vi "ComicCleaner_SM.vi"() -> ()   [LabVIEW 2023]
uses:
  <vilib>/Utility/config.llb/Write Key (Boolean).vi
  <userlib>/_OpenG.lib/array/array.llb/Remove Duplicates from 1D Array (String)__ogtk.vi
  <userlib>/_OpenG.lib/file/file.llb/Strip Path Extension - String__ogtk.vi
  <userlib>/_OpenG.lib/file/file.llb/Convert File Extension (Path)__ogtk.vi
  <vilib>/Utility/config.llb/NI_LVConfig.lvlib
panel:
  out "Destination":string
  out "Working Folder":path
  in  "Clean":bool
  in  "Clean Filename":bool=TRUE
  out "Crufted Files":string
  out "File List":string
  in  "File Path":path
  out "status":string
  in  "Quit":bool
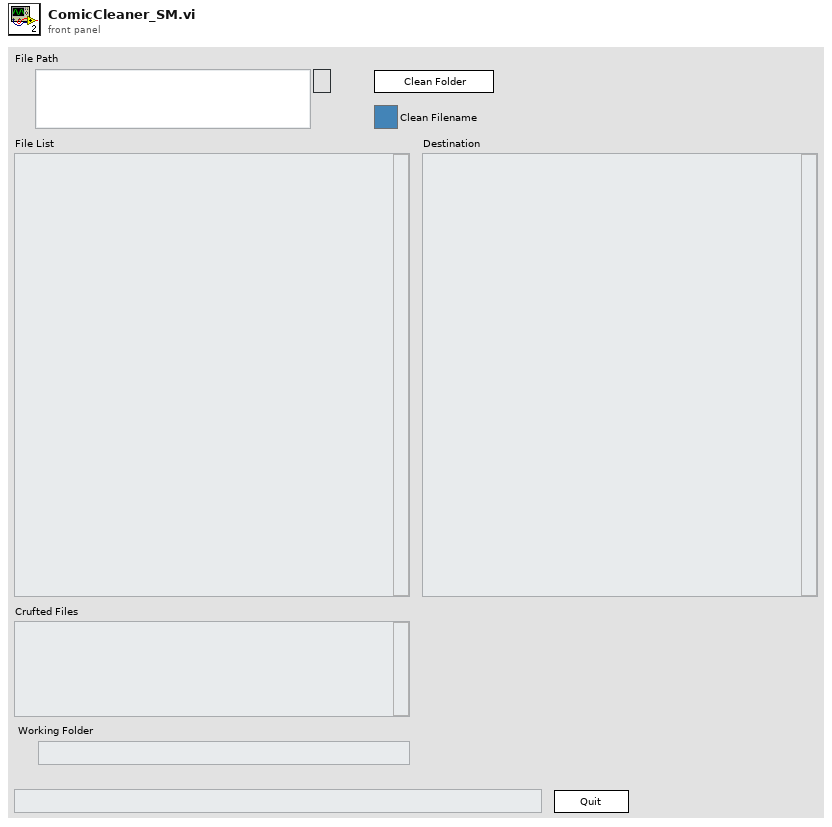
[diagram p1: front panel]
types:
  T1 = enum32{"Invalid", "Standard", "Closed", "Hidden", "Minimized", "Maximized"}
  T2 = enum32{"invalid app kind", "Development System", "Run Time System", "Student Edition", "Embedded LabVIEW", "Evaluation", "Custom"}
  T3 = enum8{"Enabled", "Disabled", "Disabled and Grayed Out"}
  T4 = cluster{"Core":cluster{"Current VI Reference":refnum<vi>, "Close Panel on Exit?":bool}, "Working Folder":path, "Known Tags":set{string}, "ini path":path, "files":path[], "current file index":i32, "deleted filenames":string[], "known found":bool, "abort":bool}
  T5 = cluster{"Current VI Reference":refnum<vi>, "Close Panel on Exit?":bool}
  T6 = typedef "NI_LVConfig.lvlib/Config Data RefNum.ctl" = refnum<k1>
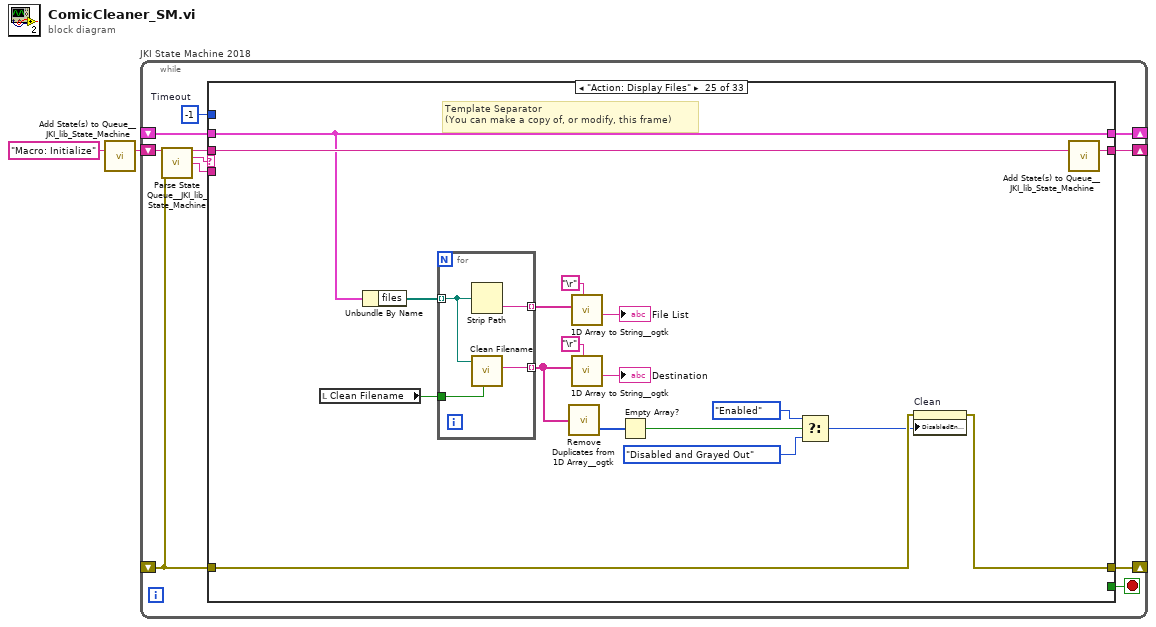
[diagram p0: block diagram]
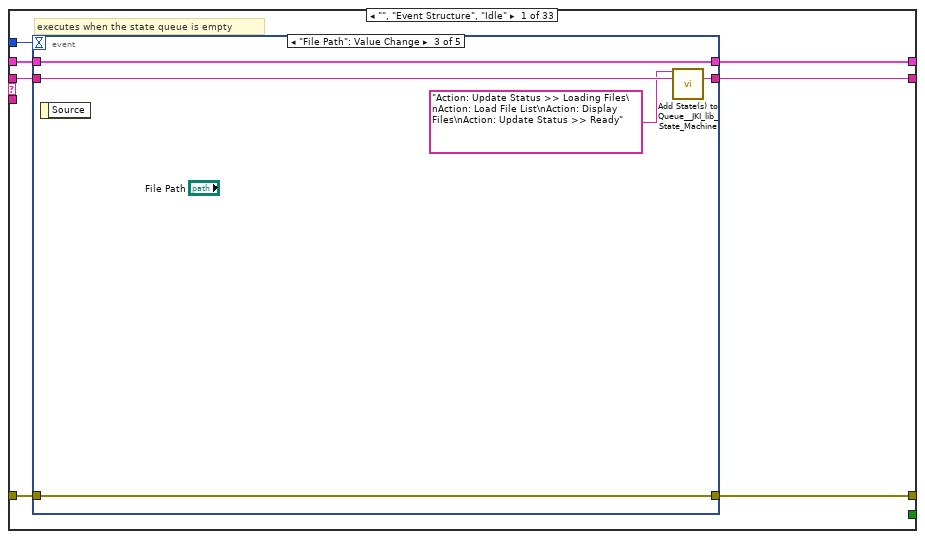
[diagram p2: hidden frame]
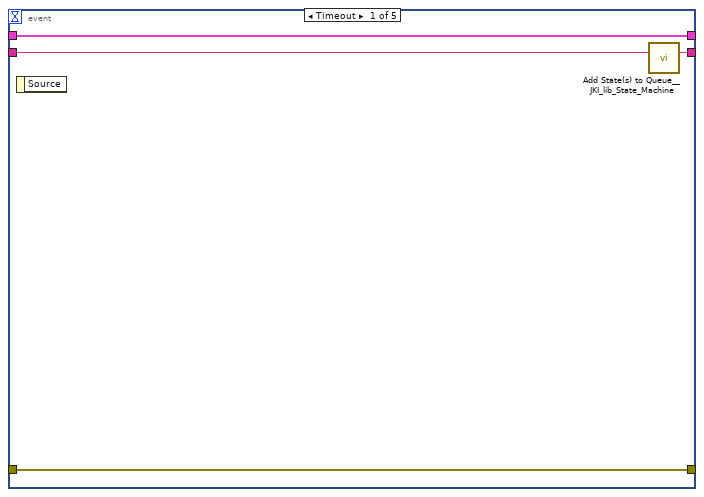
[diagram p3: hidden frame]
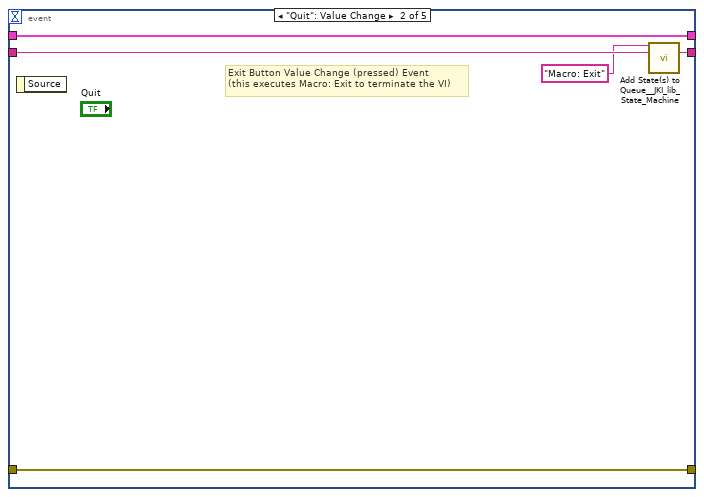
[diagram p4: hidden frame]
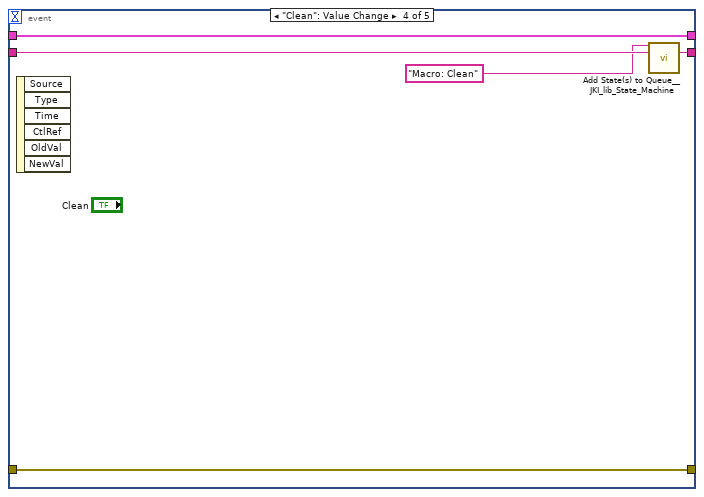
[diagram p5: hidden frame]
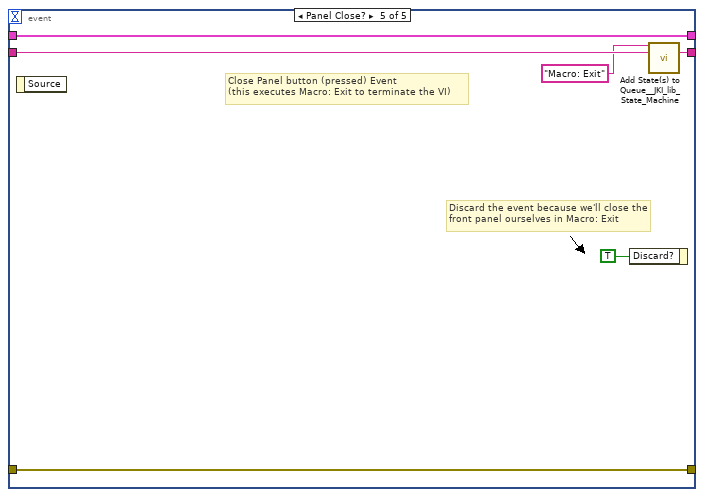
[diagram p6: hidden frame]
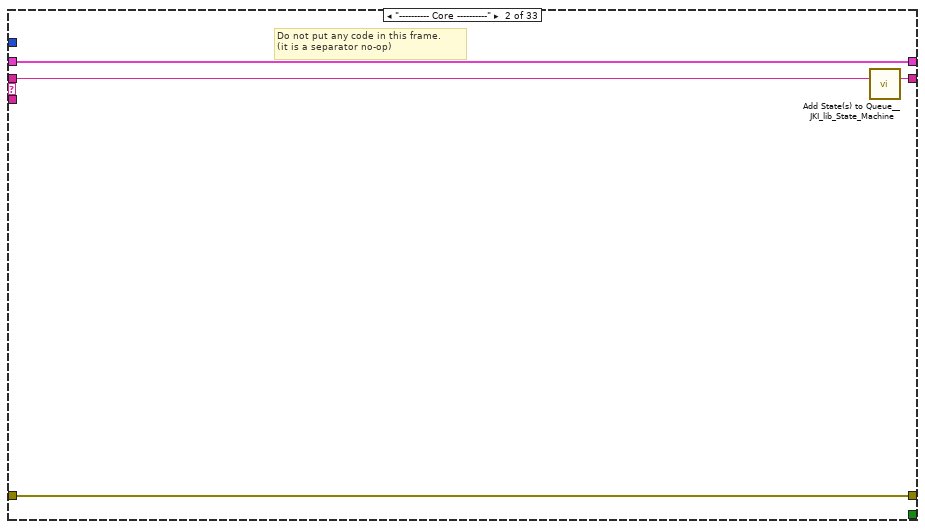
[diagram p7: hidden frame]
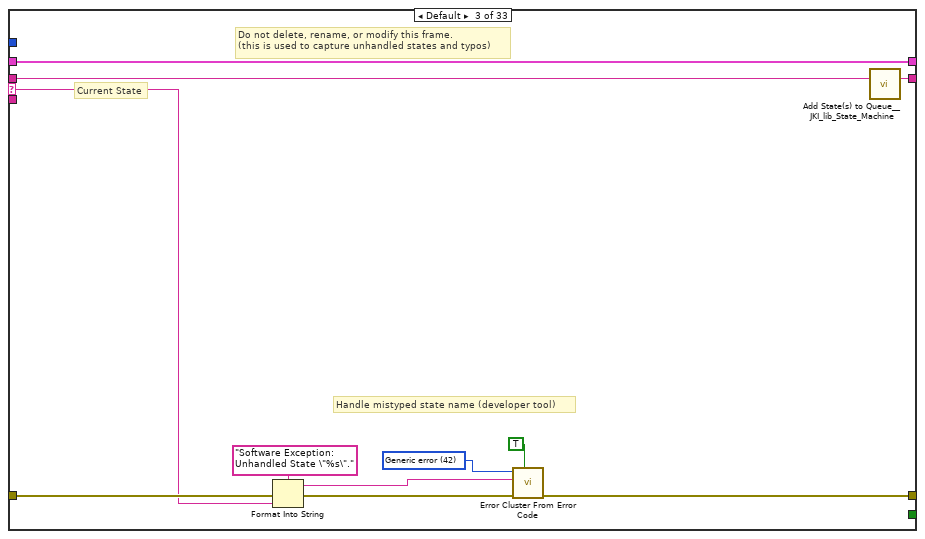
[diagram p8: hidden frame]
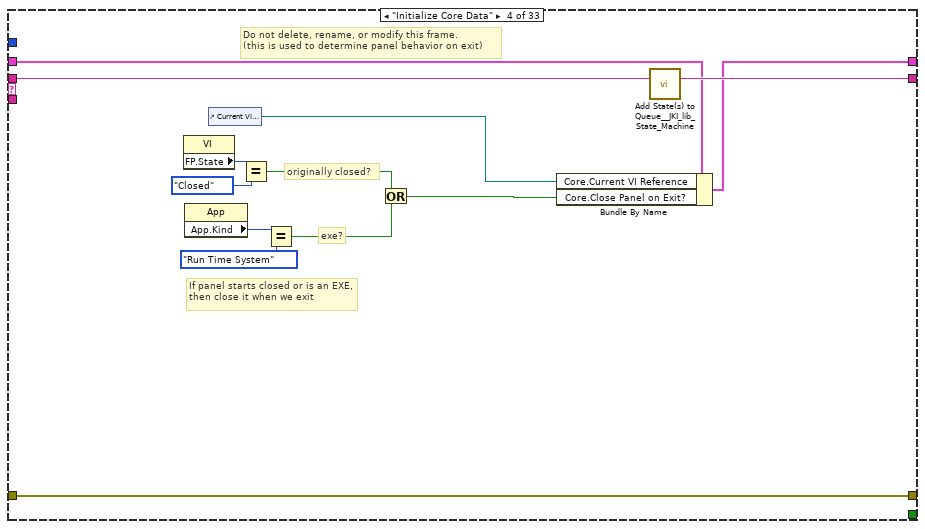
[diagram p9: hidden frame]
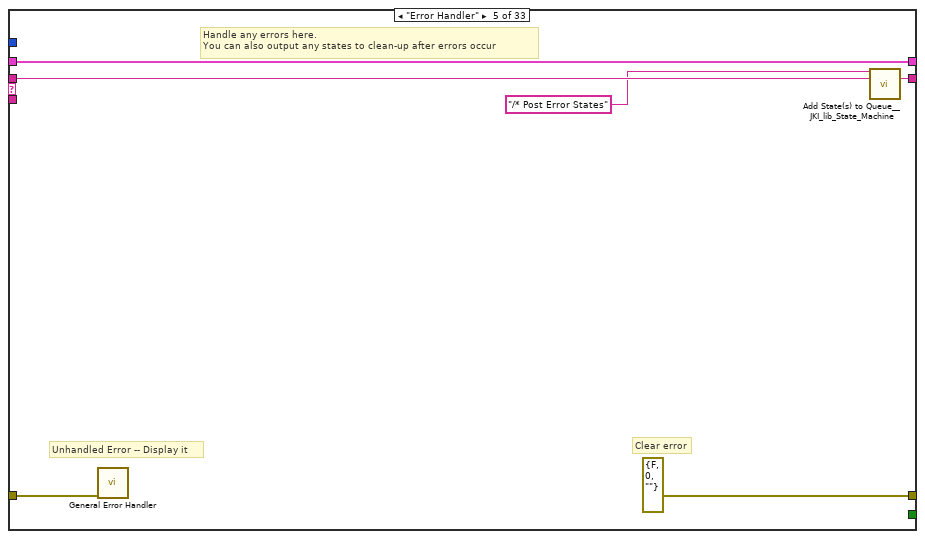
[diagram p10: hidden frame]
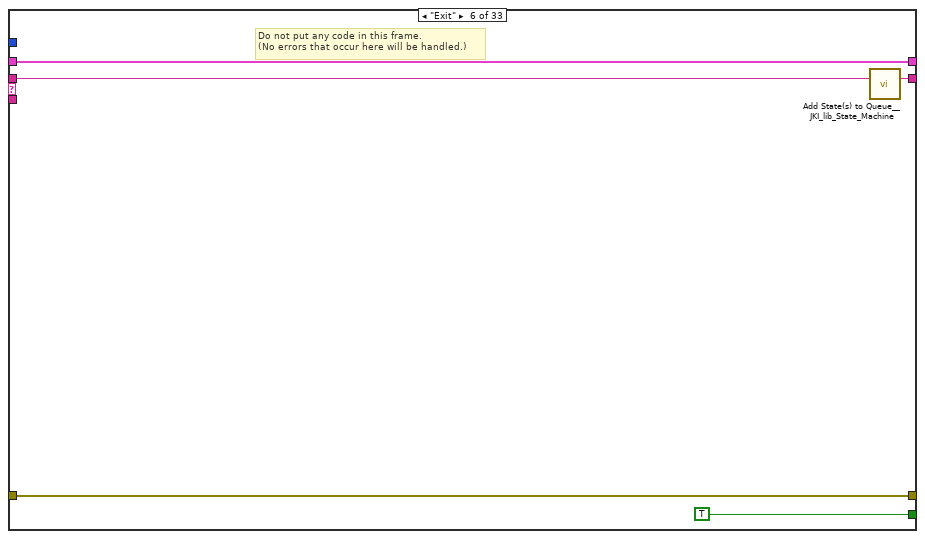
[diagram p11: hidden frame]
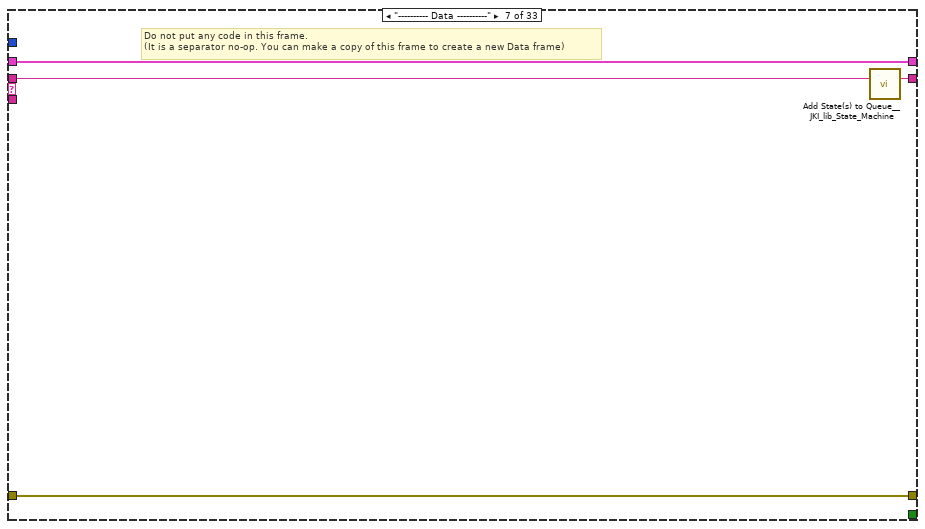
[diagram p12: hidden frame]
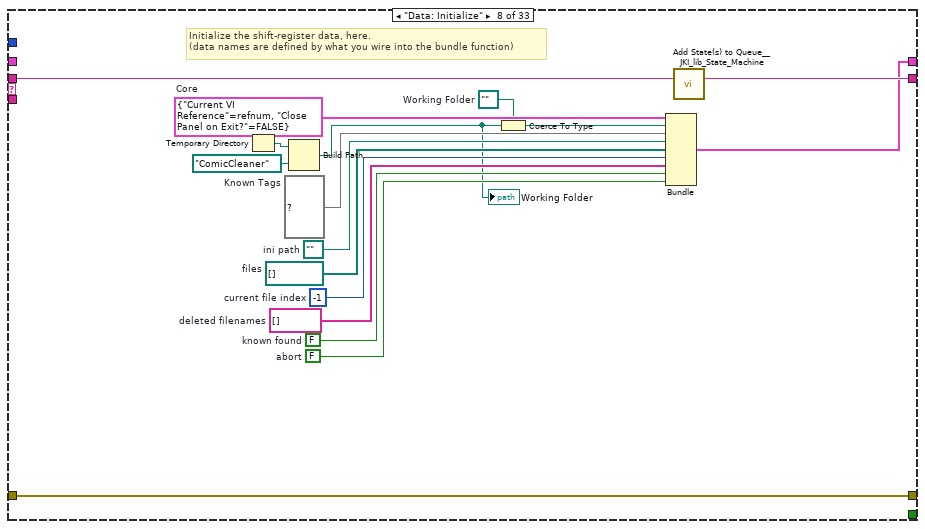
[diagram p13: hidden frame]
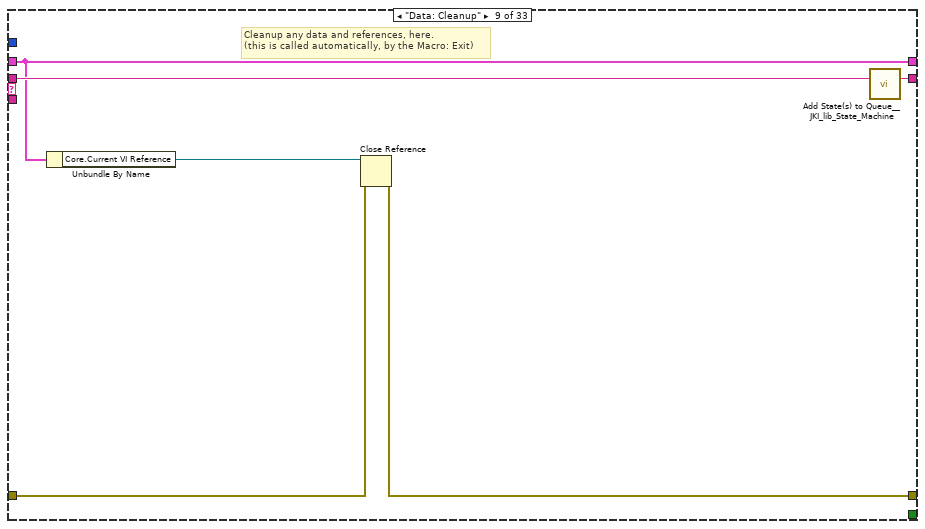
[diagram p14: hidden frame]
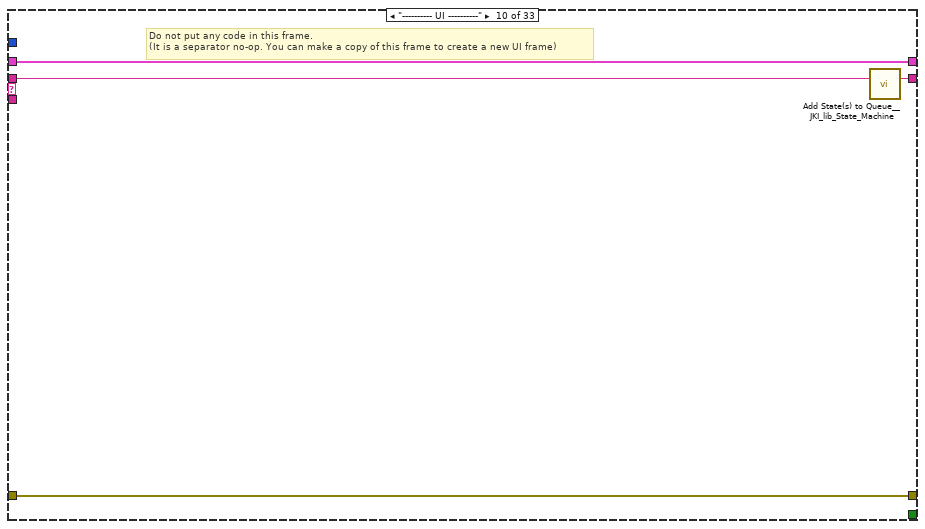
[diagram p15: hidden frame]
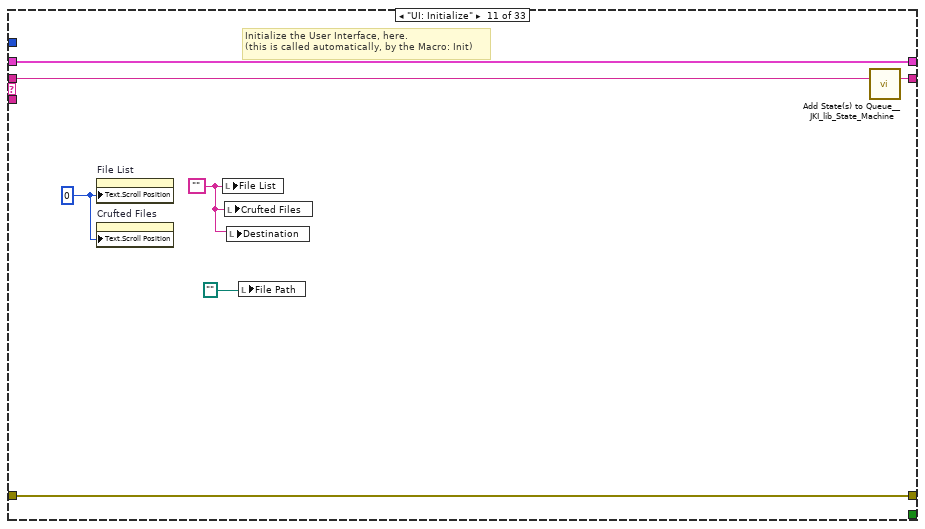
[diagram p16: hidden frame]
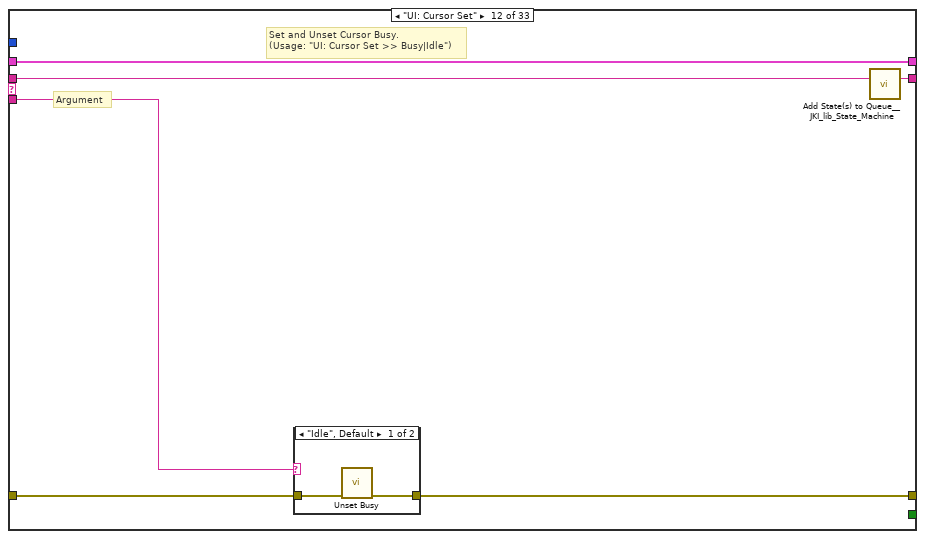
[diagram p17: hidden frame]
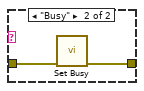
[diagram p18: hidden frame]
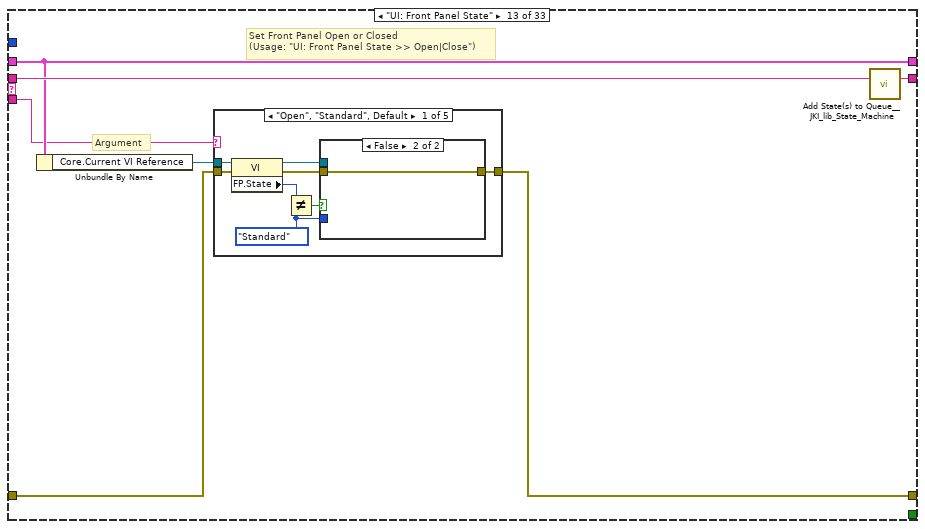
[diagram p19: hidden frame]
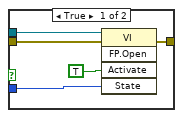
[diagram p20: hidden frame]
diagram:
  n1 = call <vilib>:"Add State(s) to Queue__JKI_lib_State_Machine.vi"("State(s) in (\"\")"="Macro: Initialize") -> ("States Out"=w2:string)  [unwired: 14 in]
  n2 = while "JKI State Machine 2018" {
    shift-right: [w6] -> _
    shift-left: _ -> [w5]
    shift-right: [w9] -> _
    shift-left: _ -> [w3]
    shift-right: [w8] -> _
    shift-left: w2 -> [w10]
    stop <- w7 stop-if-true
    w4 = -1  # Timeout
    n3 = call <vilib>:"Parse State Queue__JKI_lib_State_Machine.vi"("State Queue"=w10, "Error In (no error)"=w3) -> ("Remaining States"=w12:string, "Current State"=w13:string, "Arguments"=w11:string)  [unwired: 11 in]
    n4 = case shown="\"Action: Display Files\"" w13 {
      selector: w13 -> [_ _ w50 _ _ _ _ _ _ _ _ _ _ _ _ _ _ _ _ _ _ _ _ _ _ _ _ _ _ _ _ _ _]
      tunnel: w12 -> [w20 w49 w54 w73 w79 w84 w88 w105 w111 w115 w122 w128 w139 w208 w217 w239 w249 w253 w257 w267 w288 w307 w312 w325 w353 w361 w378 w388 w411 w433 w472 w508 w566]
      tunnel: w11 -> [_ _ _ _ _ _ _ _ _ _ _ w123 w133 _ _ _ _ _ _ _ _ w296 w308 _ _ _ _ _ _ _ _ _ _]
      tunnel: w5 -> [w18 w46 w52 w66 w76 w82 w85 _ w106 w112 w120 w126 w135 w205 w211 w236 w246 w250 w254 w259 w276 w304 w309 w319 w351 w358 w364 w381 w404 w427 w462 w496 w542]
      tunnel: [w17 w47 w56 w70 errorcluster {"status"=FALSE, "code"=0, "source"=""} ("error out") w81 w86 w102 w107 w113 w119 w124 w136 w206 w215 w237 w247 w251 w255 w260 w272 w292 w310 w314 w340 w359 w362 w379 w402 w428 w463 w499 w544] -> w9
      tunnel: w3 -> [w16 w47 w55 w70 w75 w81 w86 w102 w108 w113 w119 w125 w137 w206 w215 w237 w247 w251 w255 w265 w271 w293 w310 w320 w341 w359 w363 w380 w403 w429 w469 w504 w562]
      tunnel: [w19 w48 w53 w72 w78 w83 w87 w104 w110 w114 w121 w127 w138 w207 w216 w238 w248 w252 w256 w266 w287 w306 w311 w324 w352 w360 w377 w387 w410 w432 w471 w507 w565] -> w8
      tunnel: [_ _ _ _ _ TRUE _ _ _ _ _ _ _ _ _ _ _ _ _ _ _ _ _ _ _ _ _ _ _ _ _ _ _] -> w7
      tunnel: [w15 w46 w52 w71 w76 w82 w85 w103 w106 w112 w120 w126 w135 w205 w210 w236 w246 w250 w254 w259 w275 w305 w309 w318 w351 w358 w364 w381 w404 w426 w461 w494 w541] -> w6
      tunnel: w4 -> [w14 _ _ _ _ _ _ _ _ _ _ _ _ _ _ _ _ _ _ _ _ _ _ _ _ _ _ _ _ _ _ _ _]
      frame "", "Event Structure", "Idle" {
        # "executes when the state queue is empty"
        n5 = event shown="[2] \"File Path\": Value Change" {
          selector: _ -> [_ _ _ _ _]
          dyn-events: _ -> [_ _ _ _ _]
          timeout: w14 -> [_ _ _ _ _]
          tunnel: w20 -> [w24 w29 w34 w39 w45]
          tunnel: [w23 w28 w33 w38 w44] -> w19
          tunnel: w18 -> [w21 w26 w31 w36 w42]
          tunnel: [w22 w27 w32 w37 w43] -> w17
          tunnel: w16 -> [w22 w27 w32 w37 w43]
          tunnel: [w21 w26 w31 w36 w42] -> w15
          event Timeout {
            n6 = event-data() -> ()  [unwired: 1 in, 1 out]
            n7 = call <vilib>:"Add State(s) to Queue__JKI_lib_State_Machine.vi"("State(s) in (\"\")"=w24) -> ("States Out"=w23:string)  [unwired: 14 in]
          }
          event "Quit": Value Change {
            # "Exit Button Value Change (pressed) Event\n(this executes Macro: Exit to terminate the VI)"
            n8 = event-data() -> ()  [unwired: 1 in, 1 out]
            n9 = call <vilib>:"Add State(s) to Queue__JKI_lib_State_Machine.vi"("State(s) in Front (\"\")"="Macro: Exit", "State(s) in (\"\")"=w29) -> ("States Out"=w28:string)  [unwired: 13 in]
          }
          event "File Path": Value Change {
            n10 = event-data() -> ()  [unwired: 1 in, 1 out]
            n11 = call <vilib>:"Add State(s) to Queue__JKI_lib_State_Machine.vi"("State(s) in Front (\"\")"="Action: Update Status >> Loading Files\nAction: Load File List\nAction: Display Files\nAction: Update Status >> Ready", "State(s) in (\"\")"=w34) -> ("States Out"=w33:string)  [unwired: 13 in]
          }
          event "Clean": Value Change {
            n12 = event-data() -> ()  [unwired: 1 in, 6 out]
            n13 = call <vilib>:"Add State(s) to Queue__JKI_lib_State_Machine.vi"("State(s) in Front (\"\")"="Macro: Clean", "State(s) in (\"\")"=w39) -> ("States Out"=w38:string)  [unwired: 13 in]
          }
          event Panel Close? {
            # "Discard the event because we'll close the front panel ourselves in Macro: Exit"
            # "Close Panel button (pressed) Event\n(this executes Macro: Exit to terminate the VI)"
            n14 = event-data() -> ()  [unwired: 1 in, 1 out]
            n15 = event-data("Discard?"=TRUE) -> ()  [unwired: 1 in, 1 out]
            n16 = call <vilib>:"Add State(s) to Queue__JKI_lib_State_Machine.vi"("State(s) in Front (\"\")"="Macro: Exit", "State(s) in (\"\")"=w45) -> ("States Out"=w44:string)  [unwired: 13 in]
          }
        }
      }
      frame "---------- Core ----------" {
        # "Do not put any code in this frame.\n(it is a separator no-op)"
        n17 = call <vilib>:"Add State(s) to Queue__JKI_lib_State_Machine.vi"("State(s) in (\"\")"=w49) -> ("States Out"=w48:string)  [unwired: 14 in]
      }
      frame Default {
        w59 = 42 items=["No error", "Argument error", "Memory is full", "Out of zone", "End of file", "File already open", "Generic file I/O error", "File not found", "File permission error", "Disk is full", "Duplicate path", "Too many files open", "System feature not enabled", "Resource file not found", "Cannot add resource", "Resource not found", "Image not found", "Image memory error", "Pen does not exist", "Config type invalid", "Config token not found", "Config parse error", "Config memory error", "Bad external code format", "Bad external code offset", "External code not present", "Null window", "Destroy window error", "Null menu", "Print aborted", "Bad print record", "Print driver error", "Windows error during printing", "Memory error during printing", "Print dialog error", "Generic print error", "Invalid device refnum", "Device not found", "Device parameter error", "Device unit error", "Cannot open device", "Device call aborted", "Generic error", "Cancelled by user", "Object ID too low", "Object ID too high", "Object not in heap", "Unknown heap", "Unknown object (invalid DefProc)", "Unknown object (DefProc not in table)", "Message out of range", "Invalid (null) method", "Unknown message", "Manager call not supported", "Bad address", "Network operation in progress", "Network operation timed out", "Connection is busy", "Network attribute not supported", "Network error", "Address in use", "System out of memory", "Connection aborted", "Connection refused", "Not connected", "Already connected", "Connection closed", "Initialization error (interapplication manager)", "Bad occurrence", "Wait on unbound occurrence handler", "Occurrence queue overflow", "Datalog type conflict", "Unused", "Unrecognized type (interapplication manager)", "Memory corrupt", "Failed to make temporary DLL", "Old CIN version", "Drag socket not found", "Failed to load drop-object", "Failed to register OLE object", "Failed to release OLE object", "Format specifier type mismatch", "Unknown format specifier", "Too few format specifiers", "Too many format specifiers", "Scan failed", "Newer CIN version", "Error converting to variant", "Runtime menu error", "Password tampered", "Variant attribute not found", "Incompatible variant data type", "Event data is not available", "Event Store is not present", "Occurrence is not found", "Event Queue is not created", "Event info is not available", "Refnum passed is NULL", "Error retrieving Class GUID", "Error retrieving CoClass GUID", "Error retrieving TypeLib GUID.", "Bad built application magic bytes.", "Specific driver is different from the specific driver associated with the Logical Name.", "There is no session opened to the class driver.", "Max Error", "MAX - Error with config objects", "MAX - Error loading configuration", "MAX - Group not supported"]
        # "Current State"
        # "Do not delete, rename, or modify this frame.\n(this is used to capture unhandled states and typos)"
        # "Handle mistyped state name (developer tool)"
        n18 = Format Into String(format string="Software Exception: Unhandled State \"%s\"." ("message"), error in=w55, w50) -> (resulting string=w58:string, error out=w57:errorcluster)  [unwired: 1 in]
        n19 = call <vilib>:"Error Cluster From Error Code.vi"("show call chain? (False)"=TRUE, "error in (no error)"=w57, "error message (\"\")"=w58, "error code (0)"=w59) -> ("error out"=w56:errorcluster)  [unwired: 5 in]
        n20 = call <vilib>:"Add State(s) to Queue__JKI_lib_State_Machine.vi"("State(s) in (\"\")"=w54) -> ("States Out"=w53:string)  [unwired: 14 in]
      }
      frame "Initialize Core Data" {
        # "Do not delete, rename, or modify this frame.\n(this is used to determine panel behavior on exit)"
        # "originally closed?"
        # "exe?"
        # "If panel starts closed or is an EXE, then close it when we exit"
        n21 = property class="VI"() -> ("FP.State"=w63:T1)  [unwired: 2 in, 2 out]
        n22 = property class="App"() -> ("App.Kind"=w69:T2)  [unwired: 2 in, 2 out]
        n23 = control-ref of="Current VI Reference"() -> (w64:refnum<vi>)
        n24 = Equal?(x=w63, y=T1."Closed" ("Front Panel Window:State")) -> (x = y?=w61:bool)
        n25 = Equal?(x=w69, y=T2."Run Time System" ("Application:Kind")) -> (x = y?=w67:bool)
        n26 = Or(x=w61, y=w67) -> (x .or. y?=w65:bool)
        n27 = Bundle By Name(cluster=w66, "Core.Current VI Reference"=w64, "Core.Close Panel on Exit?"=w65) -> (w71:T4)
        n28 = call <vilib>:"Add State(s) to Queue__JKI_lib_State_Machine.vi"("State(s) in (\"\")"=w73) -> ("States Out"=w72:string)  [unwired: 14 in]
      }
      frame "Error Handler" {
        # "Unhandled Error -- Display it"
        # "Handle any errors here.\nYou can also output any states to clean-up after errors occur"
        # "Clear error"
        n29 = call <vilib>:"General Error Handler.vi"("error in (no error)"=w75) -> ()  [unwired: 10 in, 5 out]
        n30 = call <vilib>:"Add State(s) to Queue__JKI_lib_State_Machine.vi"("State(s) in Front (\"\")"="/* Post Error States", "State(s) in (\"\")"=w79) -> ("States Out"=w78:string)  [unwired: 13 in]
      }
      frame "Exit" {
        # "Do not put any code in this frame.\n(No errors that occur here will be handled.)"
        n31 = call <vilib>:"Add State(s) to Queue__JKI_lib_State_Machine.vi"("State(s) in (\"\")"=w84) -> ("States Out"=w83:string)  [unwired: 14 in]
      }
      frame "---------- Data ----------" {
        # "Do not put any code in this frame.\n(It is a separator no-op. You can make a copy of this frame to create a new Data frame)"
        n32 = call <vilib>:"Add State(s) to Queue__JKI_lib_State_Machine.vi"("State(s) in (\"\")"=w88) -> ("States Out"=w87:string)  [unwired: 14 in]
      }
      frame "Data: Initialize" {
        w90 = FALSE  # abort
        w91 = FALSE  # known found
        w92 = string[] []  # deleted filenames
        w93 = -1  # current file index
        w98 = path[] []  # files
        w99 = path ""  # ini path
        w100 = set{string} {}  # Known Tags
        w94 = path ""  # Working Folder
        w101 = T5 {"Current VI Reference"=refnum, "Close Panel on Exit?"=FALSE}  # Core
        # "Initialize the shift-register data, here.\n(data names are defined by what you wire into the bundle function)"
        n33 = Temporary Directory() -> (w97:path)
        n34 = Build Path(base path=w97, name or relative path=path "ComicCleaner") -> (appended path=w89:path)
        "Working Folder" <- w89
        n35 = Coerce To Type(0:w89, 1:w94) -> (2:w95:path)
        n36 = Bundle("Core"=w101, "Working Folder"=w95, "Known Tags"=w100, "ini path"=w99, "files"=w98, "current file index"=w93, "deleted filenames"=w92, "known found"=w91, "abort"=w90) -> (w103:T4)  [unwired: 1 in]
        n37 = call <vilib>:"Add State(s) to Queue__JKI_lib_State_Machine.vi"("State(s) in (\"\")"=w105) -> ("States Out"=w104:string)  [unwired: 14 in]
      }
      frame "Data: Cleanup" {
        # "Cleanup any data and references, here.\n(this is called automatically, by the Macro: Exit)"
        n38 = Unbundle By Name(w106) -> ("Core.Current VI Reference"=w109:refnum<vi>)
        n39 = Close Reference(reference=w109, error in (no error)=w108) -> (error out=w107:errorcluster)
        n40 = call <vilib>:"Add State(s) to Queue__JKI_lib_State_Machine.vi"("State(s) in (\"\")"=w111) -> ("States Out"=w110:string)  [unwired: 14 in]
      }
      frame "---------- UI ----------" {
        # "Do not put any code in this frame.\n(It is a separator no-op. You can make a copy of this frame to create a new UI frame)"
        n41 = call <vilib>:"Add State(s) to Queue__JKI_lib_State_Machine.vi"("State(s) in (\"\")"=w115) -> ("States Out"=w114:string)  [unwired: 14 in]
      }
      frame "UI: Initialize" {
        w118 = u32 0 ("Text.Scroll Position")
        w116 = ""
        # "Initialize the User Interface, here.\n(this is called automatically, by the Macro: Init)"
        n42 = property on="File List" class="Str"("Text.Scroll Position"=w118) -> ()  [unwired: 2 in, 2 out]
        n43 = property on="Crufted Files" class="Str"("Text.Scroll Position"=w118) -> ()  [unwired: 2 in, 2 out]
        n44 = local write "File List"(w116) -> ()
        n45 = local write "Crufted Files"(w116) -> ()
        n46 = local write "Destination"(w116) -> ()
        n47 = local write "File Path"(path "") -> ()
        n48 = call <vilib>:"Add State(s) to Queue__JKI_lib_State_Machine.vi"("State(s) in (\"\")"=w122) -> ("States Out"=w121:string)  [unwired: 14 in]
      }
      frame "UI: Cursor Set" {
        # "Argument"
        # "Set and Unset Cursor Busy.\n(Usage: \"UI: Cursor Set >> Busy|Idle\")"
        n49 = case shown="\"Idle\", Default" w123 {
          tunnel: w125 -> [w130 w132]
          tunnel: [w129 w131] -> w124
          frame "Idle", Default {
            n50 = call <vilib>:"Unset Busy.vi"("error in (no error)"=w130) -> ("error out"=w129:errorcluster)  [unwired: 10 in]
          }
          frame "Busy" {
            n51 = call <vilib>:"Set Busy.vi"("error in (no error)"=w132) -> ("error out"=w131:errorcluster)  [unwired: 9 in, 1 out]
          }
        }
        n52 = call <vilib>:"Add State(s) to Queue__JKI_lib_State_Machine.vi"("State(s) in (\"\")"=w128) -> ("States Out"=w127:string)  [unwired: 14 in]
      }
      frame "UI: Front Panel State" {
        # "Argument"
        # "Set Front Panel Open or Closed\n(Usage: \"UI: Front Panel State >> Open|Close\")"
        n53 = Unbundle By Name(w135) -> ("Core.Current VI Reference"=w134:refnum<vi>)
        n54 = case shown="\"Open\", \"Standard\", Default" w133 {
          tunnel: w137 -> [w145 w160 w171 w184 w197]
          tunnel: [w147 w161 w173 w186 w199] -> w136
          tunnel: w134 -> [w146 w158 w172 w185 w198]
          frame "Open", "Standard", Default {
            w140 = T1."Standard" ("State")
            n55 = property class="VI"(reference=w146, error in=w145) -> (reference out=w143:refnum<vi>, error out=w144:errorcluster, "FP.State"=w142:T1)
            n56 = Not Equal?(x=w142, y=w140) -> (x != y?=w141:bool)
            n57 = case shown="False" w141 {
              tunnel: [w151 w153] -> w147
              tunnel: w144 -> [w150 w153]
              tunnel: w143 -> [w149 _]
              tunnel: w140 -> [w148 _]
              frame True {
                n58 = invoke class="VI" method="FP.Open"(reference=w149, error in=w150, "Activate"=TRUE, "State"=w148) -> (error out=w151:errorcluster)  [unwired: 1 in, 4 out]
              }
              frame False {
              }
            }
          }
          frame "Close", "Closed" {
            n59 = property class="VI"(reference=w158, error in=w160) -> (reference out=w157:refnum<vi>, error out=w159:errorcluster, "FP.State"=w155:T1)
            n60 = Not Equal?(x=w155, y=T1."Closed" ("Front Panel Window:State")) -> (x != y?=w154:bool)
            n61 = case shown="True" w154 {
              tunnel: [w162 w165] -> w161
              tunnel: w159 -> [w162 w164]
              tunnel: w157 -> [_ w163]
              frame False {
              }
              frame True {
                n62 = invoke class="VI" method="FP.Close"(reference=w163, error in=w164) -> (error out=w165:errorcluster)  [unwired: 1 in, 2 out]
              }
            }
          }
          frame "Hidden", "Hide" {
            w166 = T1."Hidden" ("State")
            n63 = property class="VI"(reference=w172, error in=w171) -> (reference out=w169:refnum<vi>, error out=w170:errorcluster, "FP.State"=w168:T1)
            n64 = Not Equal?(x=w168, y=w166) -> (x != y?=w167:bool)
            n65 = case shown="True" w167 {
              tunnel: [w177 w178] -> w173
              tunnel: w170 -> [w176 w178]
              tunnel: w169 -> [w175 _]
              tunnel: w166 -> [w174 _]
              frame True {
                n66 = invoke class="VI" method="FP.Open"(reference=w175, error in=w176, "State"=w174) -> (error out=w177:errorcluster)  [unwired: 2 in, 4 out]
              }
              frame False {
              }
            }
          }
          frame "Minimize", "Minimized" {
            w179 = T1."Minimized" ("State")
            n67 = property class="VI"(reference=w185, error in=w184) -> (reference out=w182:refnum<vi>, error out=w183:errorcluster, "FP.State"=w181:T1)
            n68 = Not Equal?(x=w181, y=w179) -> (x != y?=w180:bool)
            n69 = case shown="True" w180 {
              tunnel: [w190 w191] -> w186
              tunnel: w183 -> [w189 w191]
              tunnel: w182 -> [w188 _]
              tunnel: w179 -> [w187 _]
              frame True {
                n70 = invoke class="VI" method="FP.Open"(reference=w188, error in=w189, "State"=w187) -> (error out=w190:errorcluster)  [unwired: 2 in, 4 out]
              }
              frame False {
              }
            }
          }
          frame "Maximize", "Maximized" {
            w192 = T1."Maximized" ("State")
            n71 = property class="VI"(reference=w198, error in=w197) -> (reference out=w195:refnum<vi>, error out=w196:errorcluster, "FP.State"=w194:T1)
            n72 = Not Equal?(x=w194, y=w192) -> (x != y?=w193:bool)
            n73 = case shown="True" w193 {
              tunnel: [w203 w204] -> w199
              tunnel: w196 -> [w202 w204]
              tunnel: w195 -> [w201 _]
              tunnel: w192 -> [w200 _]
              frame True {
                n74 = invoke class="VI" method="FP.Open"(reference=w201, error in=w202, "State"=w200) -> (error out=w203:errorcluster)  [unwired: 2 in, 4 out]
              }
              frame False {
              }
            }
          }
        }
        n75 = call <vilib>:"Add State(s) to Queue__JKI_lib_State_Machine.vi"("State(s) in (\"\")"=w139) -> ("States Out"=w138:string)  [unwired: 14 in]
      }
      frame "---------- Macro ----------" {
        # "Do not put any code in this frame.\n(It is a separator no-op. You can make a copy of this frame to create a new Macro frame)"
        n76 = call <vilib>:"Add State(s) to Queue__JKI_lib_State_Machine.vi"("State(s) in (\"\")"=w208) -> ("States Out"=w207:string)  [unwired: 14 in]
      }
      frame "Macro: Clean" {
        n77 = Unbundle By Name(w211) -> ("files"=w213:path[], "current file index"=w212:i32, "abort"=w214:bool)
        n78 = case shown="False" w214 {
          tunnel: w213 -> [w225 _]
          tunnel: w212 -> [w224 _]
          tunnel: w211 -> [w221 w234]
          tunnel: [w219 w234] -> w210
          tunnel: [w218 _] -> w209
          frame False {
            n79 = Array Size(array=w225) -> (size(s)=w223:i32)
            n80 = Increment(x=w224) -> (x+1=w220:i32)
            n81 = Equal?(x=w223, y=w220) -> (x = y?=w222:bool)
            n82 = case shown="False" w222 {
              tunnel: w221 -> [w229 w232]
              tunnel: w220 -> [w228 _]
              tunnel: [w227 w230] -> w219
              tunnel: ["Action: Clean Working Folder\nAction: Update Status >> Expanding Comic\nClean: Expand Comic\nAction: Update Status >> Removing Empty Folders\nClean: Remove Empty Folders\nAction: Update Status >> Resetting Permissions\nClean: Reset Permissions\nAction: Update Status >> Removing Cruft\nClean: Remove Cruft\nAction: Update Status >> Removing Known\nClean: Remove Known\nAction: Update Status >> Removing Unknown\nClean: Clean Unknown\nAction: Update Status >> Compressing Comic\nClean: Compress Comic\nAction: Display Files\nMacro: Clean" "Action: Update Status >> Clean operation complete. Ready"] -> w218
              frame False {
                n83 = Bundle By Name(cluster=w229, "current file index"=w228) -> (w227:T4)
              }
              frame True {
                n84 = Bundle By Name(cluster=w232, "current file index"=-1) -> (w230:T4)
              }
            }
          }
          frame True {
          }
        }
        n85 = call <vilib>:"Add State(s) to Queue__JKI_lib_State_Machine.vi"("State(s) in Front (\"\")"=w209, "State(s) in (\"\")"=w217) -> ("States Out"=w216:string)  [unwired: 13 in]
      }
      frame "Macro: Initialize" {
        # "Initialization Macro\n(This is called once, when the VI starts)"
        n86 = call <vilib>:"Add State(s) to Queue__JKI_lib_State_Machine.vi"("State(s) in Front (\"\")"="Data: Initialize\nInitialize Core Data\nUI: Initialize\nUI: Front Panel State >> Open\nAction: Update Status >> Reading Known Tags\nAction: Read Known Tags\nAction: Update Status >> Cleaning Working Directory\nAction: Clean Working Folder\nAction: Update Status >> Ready", "State(s) in (\"\")"=w239) -> ("States Out"=w238:string)  [unwired: 13 in]
      }
      frame "Macro: Exit" {
        # "Exit Macro\n(This is called once, when the VI exits)"
        n87 = Unbundle By Name(w246) -> ("Core.Close Panel on Exit?"=w245:bool)
        n88 = Select(t="UI: Front Panel State >> Close", s=w245, f="") -> (s? t:f=w242:string)
        n89 = call <vilib>:"Add State(s) to Queue__JKI_lib_State_Machine.vi"("State(s) in (\"\")"=w242, "State(s) at Back (\"\")"="Data: Cleanup\nExit") -> ("States Out"=w240:string)  [unwired: 13 in]
        n90 = call <vilib>:"Add State(s) to Queue__JKI_lib_State_Machine.vi"("State(s) in Front (\"\")"=w240, "State(s) in (\"\")"=w249) -> ("States Out"=w248:string)  [unwired: 13 in]
      }
      frame "Macro: Abort" {
        n91 = call <vilib>:"Add State(s) to Queue__JKI_lib_State_Machine.vi"("State(s) in (\"\")"=w253) -> ("States Out"=w252:string)  [unwired: 14 in]
      }
      frame "---------- Action ----------" {
        # "Template Separator\n(You can make a copy of, or modify, this frame)"
        n92 = call <vilib>:"Add State(s) to Queue__JKI_lib_State_Machine.vi"("State(s) in (\"\")"=w257) -> ("States Out"=w256:string)  [unwired: 14 in]
      }
      frame "Action: Clean Working Folder" {
        n93 = Unbundle By Name(w259) -> ("Working Folder"=w258:path)
        n94 = call <userlib>:"Create Dir if Non-Existant__ogtk.vi"("error in (no error)"=w265, "Directory Path"=w258) -> ("error out"=w261:errorcluster, "dup Directory Path"=w262:path)  [unwired: 7 in, 1 out]
        n95 = call <vilib>:"Recursive File List.vi"("error in (no error)"=w261, "Folder Path"=w262) -> ("error out"=w264:errorcluster, "All Files in Dir"=w263:path[])  [unwired: 5 in, 3 out]
        n96 = for {
          tunnel: w263 -> [w270] mode=indexing
          shift-right: [w268] -> w260
          shift-left: w264 -> [w269]
          n97 = Delete(path (use dialog)=w270, error in=w269) -> (error out=w268:errorcluster)  [unwired: 3 in, 2 out]
        }
        n98 = call <vilib>:"Add State(s) to Queue__JKI_lib_State_Machine.vi"("State(s) in (\"\")"=w267) -> ("States Out"=w266:string)  [unwired: 14 in]
      }
      frame "Action: Read Known Tags" {
        w285 = set{string} {}  # Size: 0
        n99 = Current VI's Path() -> (path=w278:path)
        n100 = Build Path(base path=w278, name or relative path=path "../Comic Cleaner.ini") -> (appended path=w273:path)
        n101 = call <vilib>:"Open Config Data.vi"("error in (no error)"=w271, "configuration file path"=w273) -> ("error out"=w279:errorcluster, "refnum"=w280:T6)  [unwired: 7 in, 1 out]
        n102 = call <vilib>:"Get Key Names.vi"("section"="KnownTags", "error in (no error)"=w279, "refnum"=w280) -> ("error out"=w282:errorcluster, "key names"=w284:string[], "refnum out"=w281:T6)  [unwired: 5 in, 1 out]
        n103 = To Lower Case(string=w284) -> (all lower case string=w286:string[])
        n104 = call <vilib>:"Close Config Data.vi"("error in (no error)"=w282, "refnum"=w281) -> ("error out"=w272:errorcluster)  [unwired: 8 in, 1 out]
        n105 = for {
          shift-right: [w291] -> w274
          shift-left: w285 -> [w290]
          tunnel: w286 -> [w289] mode=indexing
          n106 = Insert Into Set(10:w289, 11:w290) -> (3:w291:set{string})  [unwired: 1 out]
        }
        n107 = Bundle By Name(cluster=w276, "Known Tags"=w274, "ini path"=w273) -> (w275:T4)
        n108 = call <vilib>:"Add State(s) to Queue__JKI_lib_State_Machine.vi"("State(s) in (\"\")"=w288) -> ("States Out"=w287:string)  [unwired: 14 in]
      }
      frame "Action: Add Known Tag" {
        n109 = Unbundle By Name(w304) -> ("Known Tags"=w298:set{string}, "ini path"=w294:path)
        n110 = call <vilib>:"Open Config Data.vi"("error in (no error)"=w293, "configuration file path"=w294) -> ("error out"=w299:errorcluster, "refnum"=w300:T6)  [unwired: 7 in, 1 out]
        n111 = call-poly <vilib>:"Write Key.vi"("section"="KnownTags", "error in (no error)"=w299, "value"=TRUE, "key"=w296, "refnum"=w300) -> ("error out"=w302:errorcluster, "refnum out"=w303:T6)  [unwired: 4 in, 1 out]
        n112 = Insert Into Set(10:w296, 11:w298) -> (3:w297:set{string})  [unwired: 1 out]
        n113 = Bundle By Name(cluster=w304, "Known Tags"=w297) -> (w305:T4)
        n114 = call <vilib>:"Close Config Data.vi"("error in (no error)"=w302, "refnum"=w303) -> ("error out"=w292:errorcluster)  [unwired: 8 in, 1 out]
        n115 = call <vilib>:"Add State(s) to Queue__JKI_lib_State_Machine.vi"("State(s) in (\"\")"=w307) -> ("States Out"=w306:string)  [unwired: 14 in]
      }
      frame "Action: Update Status" {
        # "Your code here.\n(You can make a copy of, or modify, this frame)"
        n116 = call <vilib>:"Add State(s) to Queue__JKI_lib_State_Machine.vi"("State(s) in (\"\")"=w312) -> ("States Out"=w311:string)  [unwired: 14 in]
        "status" <- w308
      }
      frame "Action: Load File List" {
        n117 = local read "File Path"() -> (w316:path)
        n118 = File/Directory Info(path=w316, error in=w320) -> (path out=w323:path, directory=w322:bool, error out=w321:errorcluster)  [unwired: 4 out]
        n119 = case shown="True" w322 {
          tunnel: [w327 w334] -> w317
          tunnel: [w329 w333] -> w315
          tunnel: w321 -> [w329 w332]
          tunnel: w323 -> [w328 w331]
          tunnel: ["Clean File" "Clean Folder"] -> w313
          frame False {
            n120 = Build Array(w328) -> (w327:path[])
          }
          frame True {
            n121 = call <vilib>:"Recursive File List.vi"("pattern"="*.cb*", "error in (no error)"=w332, "Folder Path"=w331) -> ("error out"=w333:errorcluster, "All Files in Dir"=w334:path[])  [unwired: 4 in, 3 out]
          }
        }
        n122 = property on="Clean" class="Bool"(error in=w315, "BoolText.Text"=w313) -> (error out=w314:errorcluster)  [unwired: 1 in, 1 out]
        n123 = Bundle By Name(cluster=w319, "files"=w317) -> (w318:T4)
        n124 = call <vilib>:"Add State(s) to Queue__JKI_lib_State_Machine.vi"("State(s) in (\"\")"=w325) -> ("States Out"=w324:string)  [unwired: 14 in]
      }
      frame "Action: Display Files" {
        # "Template Separator\n(You can make a copy of, or modify, this frame)"
        n125 = local read "Clean Filename"() -> (w346:bool)
        n126 = Unbundle By Name(w351) -> ("files"=w347:path[])
        n127 = for {
          tunnel: w347 -> [w356] mode=indexing
          tunnel: [w357] -> w350 mode=indexing
          tunnel: w346 -> [w355]
          tunnel: [w354] -> w343 mode=indexing
          n128 = Strip Path(path=w356) -> (name=w357:string)  [unwired: 1 out]
          n129 = call "Clean Filename.vi"("Clean Filename?"=w355, "Filepath in"=w356) -> ("Filename out"=w354:string)  [unwired: 8 in, 1 out]
        }
        n130 = call-poly <userlib>:"Remove Duplicates from 1D Array__ogtk.vi"("Input Array"=w343) -> ("indices of removed elements"=w342:i32[])  [unwired: 1 out]
        n131 = call <userlib>:"1D Array to String__ogtk.vi"("delimiter (Tab)"="\r", "Array of Strings"=w350) -> ("delimited string"=→"File List":string)  [unwired: 9 in]
        n132 = call <userlib>:"1D Array to String__ogtk.vi"("delimiter (Tab)"="\r", "Array of Strings"=w343) -> ("delimited string"=→"Destination":string)  [unwired: 9 in]
        n133 = Empty Array?(array=w342) -> (empty?=w339:bool)
        n134 = Select(t=T3."Enabled" ("Disabled"), s=w339, f=T3."Disabled and Grayed Out" ("Disabled")) -> (s? t:f=w336:T3)
        n135 = property on="Clean" class="Bool"(error in=w341, "DisabledEnum"=w336) -> (error out=w340:errorcluster)  [unwired: 1 in, 1 out]
        n136 = call <vilib>:"Add State(s) to Queue__JKI_lib_State_Machine.vi"("State(s) in (\"\")"=w353) -> ("States Out"=w352:string)  [unwired: 14 in]
      }
      frame "---------- Clean ----------" {
        # "Template Separator\n(You can make a copy of, or modify, this frame)"
        n137 = call <vilib>:"Add State(s) to Queue__JKI_lib_State_Machine.vi"("State(s) in (\"\")"=w361) -> ("States Out"=w360:string)  [unwired: 14 in]
      }
      frame "Clean: Expand Comic" {
        n138 = Unbundle By Name(w364) -> ("files"=w376:path[], "current file index"=w375:i32, "Working Folder"=w367:path)
        n139 = Index Array(array=w376, index=w375) -> (element=w366:path)
        n140 = call "PathToQuotedString.vi"("Path"=w367) -> ("String"=w372:string)  [unwired: 10 in]
        n141 = call "PathToQuotedString.vi"("Path"=w366) -> ("String"=w373:string)  [unwired: 10 in]
        n142 = Format Into String(format string="%s e %s -o%s -r", "\"C:\\Program Files\\7-Zip\\7z.exe\"" ("input 1"), w373, w372) -> (resulting string=w370:string, error out=w369:errorcluster)  [unwired: 2 in]
        n143 = call <vilib>:"System Exec.vi"("run minimized? (F)"=TRUE, "error in (no error)"=w369, "command line"=w370) -> ("error out"=w365:errorcluster)  [unwired: 5 in, 3 out]
        n144 = Merge Errors(w363, w365) -> (w362:errorcluster)
        n145 = call <vilib>:"Add State(s) to Queue__JKI_lib_State_Machine.vi"("State(s) in (\"\")"=w378) -> ("States Out"=w377:string)  [unwired: 14 in]
      }
      frame "Clean: Remove Empty Folders" {
        n146 = Unbundle By Name(w381) -> ("Working Folder"=w382:path)
        n147 = List Folder(path=w382, error in=w380) -> (path out=w386:path, folder names=w384:string[], error out=w385:errorcluster)  [unwired: 2 in, 1 out]
        n148 = Empty Array?(array=w384) -> (empty?=w383:bool)
        n149 = case shown="True" w383 {
          tunnel: w384 -> [w392 _]
          tunnel: w386 -> [w389 _]
          tunnel: w385 -> [w391 w401]
          tunnel: [w390 w401] -> w379
          frame False {
            n150 = for {
              tunnel: w392 -> [w399] mode=indexing
              tunnel: w389 -> [w400]
              shift-right: [w398] -> w390
              shift-left: w391 -> [w393]
              n151 = Build Path(base path=w400, name or relative path=w399) -> (appended path=w394:path)
              n152 = Set Permissions(7:i16 438 ("permissions"), 8:w393, 11:w394) -> (0:w397:errorcluster, 3:w396:path)  [unwired: 2 in]
              n153 = Delete(path (use dialog)=w396, error in=w397) -> (error out=w398:errorcluster)  [unwired: 3 in, 2 out]
            }
          }
          frame True {
          }
        }
        n154 = call <vilib>:"Add State(s) to Queue__JKI_lib_State_Machine.vi"("State(s) in (\"\")"=w388) -> ("States Out"=w387:string)  [unwired: 14 in]
      }
      frame "Clean: Reset Permissions" {
        n155 = Unbundle By Name(w404) -> ("Working Folder"=w406:path)
        n156 = List Folder(path=w406, error in=w403) -> (path out=w405:path, filenames=w407:string[], error out=w408:errorcluster)  [unwired: 2 in, 1 out]
        n157 = Empty Array?(array=w407) -> (empty?=w409:bool)
        n158 = case shown="False" w409 {
          tunnel: w407 -> [w415 _]
          tunnel: w405 -> [w412 _]
          tunnel: w408 -> [w414 w422]
          tunnel: [w413 w422] -> w402
          frame False {
            n159 = for {
              tunnel: w415 -> [w420] mode=indexing
              tunnel: w412 -> [w421]
              shift-right: [w417] -> w413
              shift-left: w414 -> [w418]
              n160 = Build Path(base path=w421, name or relative path=w420) -> (appended path=w416:path)
              n161 = Set Permissions(7:i16 438 ("permissions"), 8:w418, 11:w416) -> (0:w417:errorcluster)  [unwired: 2 in, 1 out]
            }
          }
          frame True {
          }
        }
        n162 = call <vilib>:"Add State(s) to Queue__JKI_lib_State_Machine.vi"("State(s) in (\"\")"=w411) -> ("States Out"=w410:string)  [unwired: 14 in]
      }
      frame "Clean: Remove Cruft" {
        # "Remove non-jpg files"
        n163 = Unbundle By Name(w427) -> ("Working Folder"=w430:path)
        n164 = for {
          shift-right: [w435] -> w428
          shift-left: w429 -> [w441]
          tunnel: string[] ["*.txt", "*.xml", "*.sfv", "*.db", "*.nfo", "*.htm", "*.sfv"] -> [w440] mode=indexing
          tunnel: [w434] -> w424 mode=concatenating
          tunnel: w430 -> [w439]
          n165 = List Folder(path=w439, pattern=w440, error in=w441) -> (filenames=w437:string[], error out=w436:errorcluster)  [unwired: 1 in, 2 out]
          n166 = Empty Array?(array=w437) -> (empty?=w438:bool)
          n167 = case shown="True" w438 {
            tunnel: w437 -> [w446 _]
            tunnel: w439 -> [w443 _]
            tunnel: w436 -> [w445 w453]
            tunnel: [w444 w453] -> w435
            tunnel: [w442 string[] []] -> w434
            frame False {
              n168 = for {
                tunnel: w446 -> [w447] mode=indexing
                tunnel: w443 -> [w450]
                shift-right: [w448] -> w444
                shift-left: w445 -> [w449]
                tunnel: [w447] -> w442 mode=indexing
                n169 = Build Path(base path=w450, name or relative path=w447) -> (appended path=w451:path)
                n170 = Delete(path (use dialog)=w451, error in=w449) -> (error out=w448:errorcluster)  [unwired: 3 in, 2 out]
              }
            }
            frame True {
            }
          }
        }
        n171 = call <userlib>:"1D Array to String__ogtk.vi"("delimiter (Tab)"="\r", "Array of Strings"=w424) -> ("delimited string"=→"Crufted Files":string)  [unwired: 9 in]
        n172 = Bundle By Name(cluster=w427, "deleted filenames"=w424) -> (w426:T4)
        n173 = call <vilib>:"Add State(s) to Queue__JKI_lib_State_Machine.vi"("State(s) in (\"\")"=w433) -> ("States Out"=w432:string)  [unwired: 14 in]
      }
      frame "Clean: Remove Known" {
        n174 = Unbundle By Name(w462) -> ("deleted filenames"=w459:string[], "Known Tags"=w465:set{string}, "Working Folder"=w470:path)
        n175 = List Folder(path=w470, error in=w469) -> (path out=w466:path, filenames=w468:string[], error out=w464:errorcluster)  [unwired: 2 in, 1 out]
        n176 = To Lower Case(string=w468) -> (all lower case string=w467:string[])
        n177 = for {
          shift-right: [w484] -> w463
          shift-left: w464 -> [w485]
          tunnel: w467 -> [w482] mode=indexing
          tunnel: w465 -> [w475]
          tunnel: w466 -> [w483]
          tunnel: [w481] -> w460 mode=indexing if=w473
          tunnel: [w473] -> w455 mode=indexing
          n178 = String Subset(string=w482, length (rest)=2 ("length (rest)")) -> (substring=w479:string)  [unwired: 1 in]
          n179 = Insert Into Set(10:w482, 11:w475) -> (2:w474:bool)  [unwired: 1 out]
          n180 = Equal?(x=w479, y="zz") -> (x = y?=w476:bool)
          n181 = Or(x=w476, y=w474) -> (x .or. y?=w477:bool)
          n182 = case shown="False" w477 {
            selector: w477 -> [w486 _]
            tunnel: w485 -> [w491 w493]
            tunnel: [w490 w493] -> w484
            tunnel: w483 -> [w489 _]
            tunnel: w482 -> [w487 w492]
            tunnel: [w486 _] -> w473
            tunnel: [w487 w492] -> w481
            frame True {
              n183 = Build Path(base path=w489, name or relative path=w487) -> (appended path=w488:path)
              n184 = Delete(path (use dialog)=w488, error in=w491) -> (error out=w490:errorcluster)  [unwired: 3 in, 2 out]
            }
            frame False {
            }
          }
        }
        n185 = Or Array Elements(Boolean array=w455) -> (logical OR=w454:bool)
        n186 = Build Array (concatenate)(w459, w460) -> (w457:string[])
        n187 = Bundle By Name(cluster=w462, "known found"=w454, "deleted filenames"=w457) -> (w461:T4)
        n188 = call <userlib>:"1D Array to String__ogtk.vi"("delimiter (Tab)"="\r", "Array of Strings"=w457) -> ("delimited string"=w456:string)  [unwired: 9 in]
        n189 = local write "Crufted Files"(w456) -> ()
        n190 = call <vilib>:"Add State(s) to Queue__JKI_lib_State_Machine.vi"("State(s) in (\"\")"=w472) -> ("States Out"=w471:string)  [unwired: 14 in]
      }
      frame "Clean: Clean Unknown" {
        n191 = Unbundle By Name(w496) -> ("known found"=w503:bool, "Working Folder"=w505:path)
        n192 = List Folder(path=w505, error in=w504) -> (path out=w498:path, filenames=w506:string[], error out=w500:errorcluster)  [unwired: 2 in, 1 out]
        n193 = call "Check Abnormal.vi"("Known Found?"=w503, "Filenames"=w506) -> ("Ignore"=w502:bool, "Filenames out"=w501:string[])  [unwired: 8 in]
        n194 = case shown="True" w502 {
          tunnel: [w515 w536] -> w499
          tunnel: w500 -> [w514 w536]
          tunnel: w498 -> [w513 _]
          tunnel: w501 -> [w517 _]
          tunnel: [w510 _] -> w497
          tunnel: [w509 _] -> w495
          frame False {
            n195 = Reverse 1D Array(array=w517) -> (reversed array=w516:string[])
            n196 = Index Array(array=w516) -> (element=w512:string)  [unwired: 1 in]
            n197 = call-poly <userlib>:"Strip Path Extension__ogtk.vi"("path"=w512) -> ("extension"=w511:string)  [unwired: 1 out]
            n198 = case shown="\"jpg\"" w511 {
              tunnel: [w518 w526] -> w515
              tunnel: w514 -> [w518 w525]
              tunnel: w513 -> [_ w524]
              tunnel: w512 -> [_ w521]
              tunnel: [_ w520] -> w510
              tunnel: [_ w519] -> w509
              frame Default {
              }
              frame "jpg" {
                n199 = Build Path(base path=w524, name or relative path=w521) -> (appended path=w523:path)
                n200 = call "Cruft Dialog.vi"("Path"=w523) -> ("Result"=w522:enum16{"Add", "Ignore", "Abort"})  [unwired: 10 in]
                n201 = case shown="\"Abort\"" w522 {
                  tunnel: w525 -> [w530 w533 w535]
                  tunnel: w521 -> [w529 _ _]
                  tunnel: [w532 w533 w535] -> w526
                  tunnel: w523 -> [w531 _ _]
                  tunnel: [w527 _ _] -> w520
                  tunnel: [_ _ TRUE] -> w519
                  frame "Add" {
                    n202 = Delete(path (use dialog)=w531, error in=w530) -> (error out=w532:errorcluster)  [unwired: 3 in, 2 out]
                    n203 = Format Into String(format string="Action: Add Known Tag >> %s", w529) -> (resulting string=w527:string)  [unwired: 2 in, 1 out]
                  }
                  frame "Ignore" {
                  }
                  frame "Abort" {
                  }
                }
              }
            }
          }
          frame True {
          }
        }
        n204 = Bundle By Name(cluster=w496, "abort"=w495) -> (w494:T4)
        n205 = call <vilib>:"Add State(s) to Queue__JKI_lib_State_Machine.vi"("State(s) in Front (\"\")"=w497, "State(s) in (\"\")"=w508) -> ("States Out"=w507:string)  [unwired: 13 in]
      }
      frame "Clean: Compress Comic" {
        # "Template Separator\n(You can make a copy of, or modify, this frame)"
        n206 = Unbundle By Name(w542) -> ("files"=w540:path[], "current file index"=w539:i32, "Working Folder"=w546:path)
        n207 = Index Array(array=w540, index=w539) -> (element=w561:path)
        n208 = Set Permissions(7:i16 438 ("permissions"), 8:w562, 11:w561) -> (0:w558:errorcluster, 3:w564:path)  [unwired: 2 in]
        n209 = Delete(path (use dialog)=w564, error in=w558) -> (deleted path=w555:path, error out=w548:errorcluster)  [unwired: 3 in, 1 out]
        n210 = Build Path(base path=w546, name or relative path="*.*") -> (appended path=w559:path)
        n211 = Array Size(array=w540) -> (size(s)=w543:i32)
        n212 = call-poly <userlib>:"Convert File Extension__ogtk.vi"("new ending (none)"="cbz", "file name"=w555) -> ("new filename"=w557:path)  [unwired: 1 out]
        n213 = call "Clean Filename.vi"("Clean Filename?"="Clean Filename", "Filepath in"=w557) -> ("Filepath out"=w538:path)  [unwired: 8 in, 1 out]
        n214 = case shown="Default" w543 {
          tunnel: w538 -> [_ w567]
          frame Default {
          }
          frame 1 {
            n215 = local write "File Path"(w567) -> ()
          }
        }
        n216 = call "PathToQuotedString.vi"("Path"=w559) -> ("String"=w545:string)  [unwired: 10 in]
        n217 = call "PathToQuotedString.vi"("Path"=w538) -> ("String"=w547:string)  [unwired: 10 in]
        n218 = Format Into String(format string="%s a -tzip %s %s", error in=w548, "\"C:\\Program Files\\7-Zip\\7z.exe\"" ("input 1"), w547, w545) -> (resulting string=w551:string, error out=w552:errorcluster)  [unwired: 1 in]
        n219 = call <vilib>:"System Exec.vi"("run minimized? (F)"=TRUE, "error in (no error)"=w552, "command line"=w551) -> ("error out"=w544:errorcluster)  [unwired: 5 in, 3 out]
        n220 = Replace Array Subset(array=w540, new element=w538, index=w539) -> (w537:path[])
        n221 = Bundle By Name(cluster=w542, "files"=w537) -> (w541:T4)
        n222 = call <vilib>:"Add State(s) to Queue__JKI_lib_State_Machine.vi"("State(s) in (\"\")"=w566) -> ("States Out"=w565:string)  [unwired: 14 in]
      }
    }
  }
